vi "DELETEGet SMO RC Type.vi"(8 "error in (no error)":errorcluster, 11 "Inst.AH2500Instrument in":refnum<class "Inst.AH2500.lvclass">) -> (0 "error out":errorcluster, 2 "Configuration.SMO.RC Type":T1=enum."STM", 3 "Inst.AH2500Instrument out":refnum<class "Inst.AH2500.lvclass">)   [LabVIEW 2019]
uses:
  <userlib>/LevyLab/RemoteControl/RemoteControl/RemoteControl.lvclass
  C:/Program Files (x86)/National Instruments/LabVIEW 2019/vi.lib/JKI/JKI SMO/SMO/SMO.lvclass
  <userlib>/LevyLab/RemoteControl/RemoteControl/Typedefs/RC Com Type--enum.ctl
  SMOs/Inst.AH2500/Inst.AH2500.lvclass
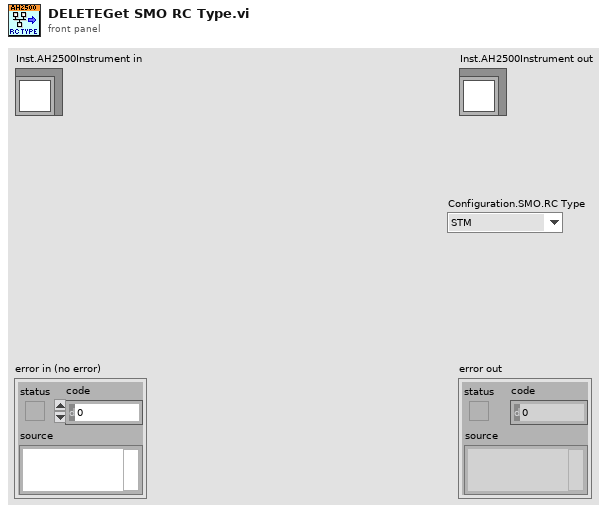
[diagram p1: front panel]
types:
  T1 = typedef "RemoteControl.lvlib/RemoteControl.lvclass/RC Com Type--enum.ctl" = enum16{"RC", "STM", "ZMQ"}
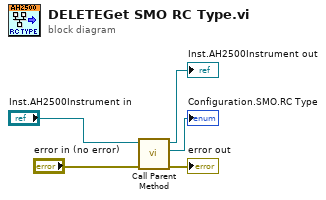
[diagram p0: block diagram]
diagram:
  n1 = call-parent "Call Parent Method"("error in (no error)"="error in (no error)", "Instrument in"="Inst.AH2500Instrument in") -> ("error out"=→"error out":errorcluster, "RemoteControl"=→"Configuration.SMO.RC Type":refnum<class "RemoteControl.lvclass">, "Instrument out"=→"Inst.AH2500Instrument out":refnum<class "Inst.AH2500.lvclass">)  [unwired: 7 in]
